vi "Td-K.vi"(0 "Blower Opening \nInput (Degrees)":dbl(slide) caption="Blower Opening (Degreees)" scale=15.0..90.0) -> (1 "K Calculated":dbl, 2 "Tau-d Calculated":dbl)   [LabVIEW 2018]
uses:
  <vilib>/Analysis/NI_AALPro.lvlib
panel:
  out "Polynomial Order \n(Fixed for Curve Fitting)":dbl=2.0
  out "K - Measurements for\nBlower Openings":dbl[](array[numeric])
  out "Tau-d Measurements for\nBlower Openings":dbl[](array[numeric])
  out "Blower Opening \nMeasurements (Degrees)":dbl[](array[numeric])
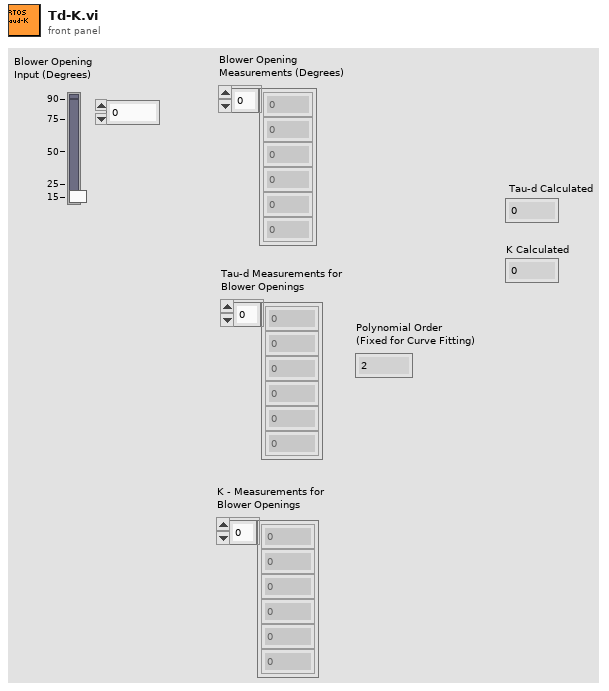
[diagram p1: front panel]
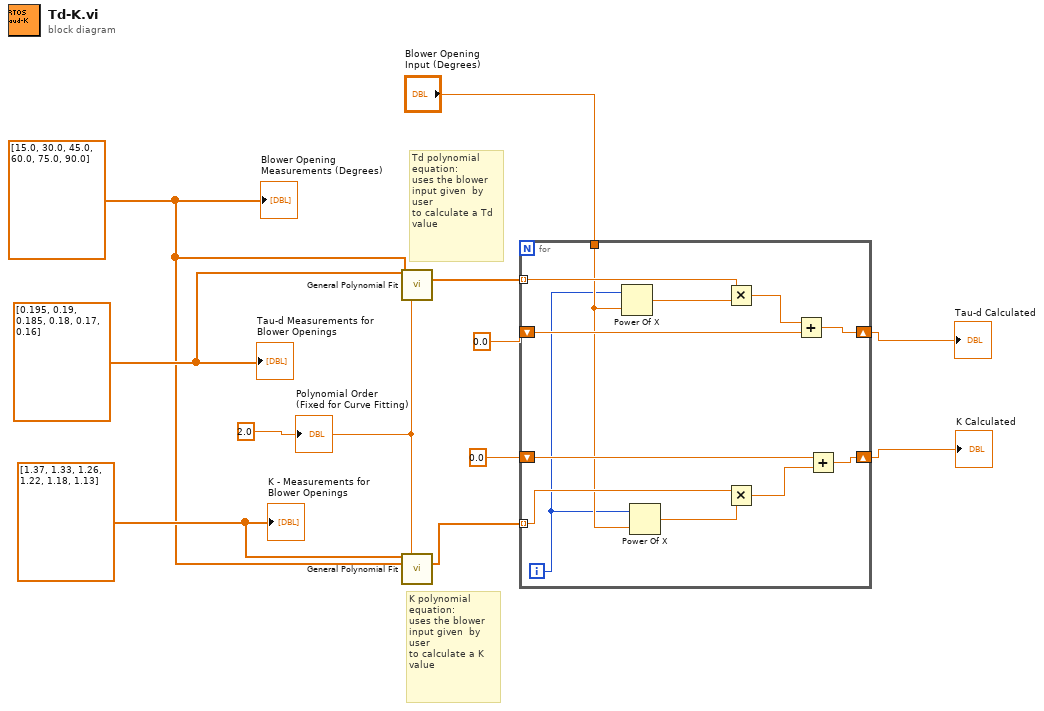
[diagram p0: block diagram]
diagram:
  w1 = 2.0
  w10 = dbl[] [1.37, 1.33, 1.26, 1.22, 1.18, 1.13]
  w11 = dbl[] [0.195, 0.19, 0.185, 0.18, 0.17, 0.16]
  w9 = dbl[] [15.0, 30.0, 45.0, 60.0, 75.0, 90.0]
  # "K polynomial equation: \nuses the blower input given  by user \nto calculate a K value"
  # "Td polynomial equation: \nuses the blower input given  by user \nto calculate a Td value"
  n1 = call <vilib>:"General Polynomial Fit.vi"("Y"=w11, "polynomial order"=w1, "X"=w9) -> ("Polynomial Coefficients"=w8:dbl[])  [unwired: 9 in, 3 out]
  n2 = call <vilib>:"General Polynomial Fit.vi"("Y"=w10, "polynomial order"=w1, "X"=w9) -> ("Polynomial Coefficients"=w7:dbl[])  [unwired: 9 in, 3 out]
  n3 = for {
    tunnel: w8 -> [w17] mode=indexing
    tunnel: w7 -> [w16] mode=indexing
    tunnel: "Blower Opening \nInput (Degrees)" -> [w13]
    shift-right: [w22] -> w3
    shift-left: 0.0 -> [w21]
    shift-right: [w23] -> w2
    shift-left: 0.0 -> [w20]
    i -> [w12]
    n4 = Power Of X(1:w13, 2:w12) -> (0:w15:dbl)
    n5 = Power Of X(1:w13, 2:w12) -> (0:w14:dbl)
    n6 = Multiply(x=w17, y=w15) -> (x*y=w18:dbl)
    n7 = Multiply(x=w16, y=w14) -> (x*y=w19:dbl)
    n8 = Add(x=w18, y=w21) -> (x+y=w22:dbl)
    n9 = Add(x=w20, y=w19) -> (x+y=w23:dbl)
  }
  "Tau-d Calculated" <- w3
  "K Calculated" <- w2
  "Blower Opening \nMeasurements (Degrees)" <- w9
  "Tau-d Measurements for\nBlower Openings" <- w11
  "K - Measurements for\nBlower Openings" <- w10
  "Polynomial Order \n(Fixed for Curve Fitting)" <- w1
